vi "FTW-ProjectItem-Tag-Set.vi"(0 "ProjectItem":refnum<vi>, 5 "Tag Name":string, 7 "Tag Value":variant, 9 "Persistent?":bool, 11 "error in":errorcluster) -> (4 "ProjectItem out":refnum<vi>, 15 "error out":errorcluster)   [LabVIEW 2012]
panel:
  # "Inputs"
  # "Outputs"
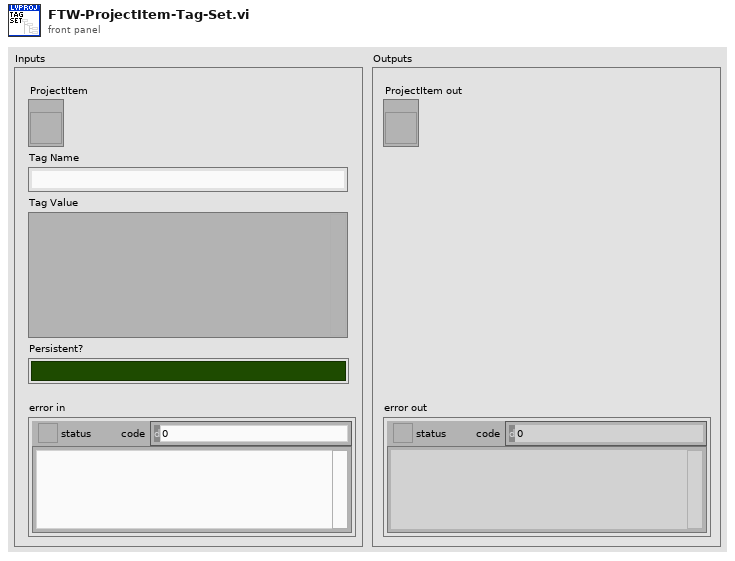
[diagram p1: front panel]
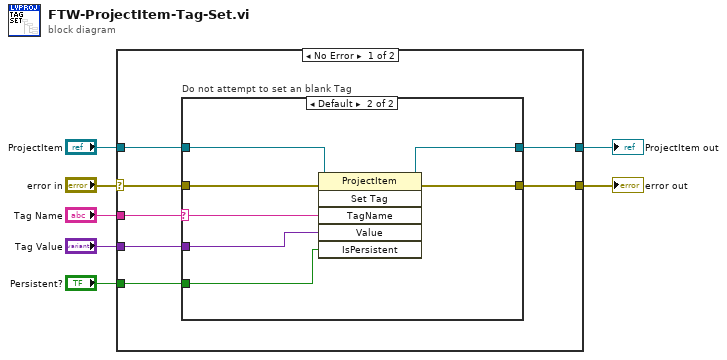
[diagram p0: block diagram]
diagram:
  n1 = case shown="No Error" "error in" {
    selector: "error in" -> [w14 w25]
    tunnel: [w13 w25] -> w7
    tunnel: "Tag Name" -> [w11 _]
    tunnel: "Tag Value" -> [w12 _]
    tunnel: "ProjectItem" -> [w10 w24]
    tunnel: "Persistent?" -> [w9 _]
    tunnel: [w8 w24] -> w1
    frame No Error {
      n2 = case "Do not attempt to set an blank Tag" shown="Default" w11 {
        selector: w11 -> [_ w20]
        tunnel: w14 -> [w16 w23]
        tunnel: [w16 w22] -> w13
        tunnel: w12 -> [_ w21]
        tunnel: w10 -> [w15 w19]
        tunnel: w9 -> [_ w18]
        tunnel: [w15 w17] -> w8
        frame "" {
        }
        frame Default {
          n3 = invoke class="ProjectItem" method="Set Tag"(reference=w19, error in=w23, "TagName"=w20, "Value"=w21, "IsPersistent"=w18) -> (reference out=w17:refnum<vi>, error out=w22:errorcluster)  [unwired: 1 in, 4 out]
        }
      }
    }
    frame Error {
    }
  }
  "error out" <- w7
  "ProjectItem out" <- w1
